vi "Lab Panel V5.22.1.vi"() -> ()   [LabVIEW 2013] (continued)
                    n2885 = Number To Fractional String(number=w5287, precision (6)=w5245) -> (F-format string=w5285:string)  [unwired: 2 in]
                    n2886 = Number To Fractional String(number=w5297, precision (6)=w5245) -> (F-format string=w5295:string)  [unwired: 2 in]
                    n2887 = Number To Fractional String(number=w5292, precision (6)=w5245) -> (F-format string=w5290:string)  [unwired: 2 in]
                    n2888 = Number To Fractional String(number=w5277, precision (6)=w5245) -> (F-format string=w5275:string)  [unwired: 2 in]
                    n2889 = Number To Fractional String(number=w5282, precision (6)=w5245) -> (F-format string=w5280:string)  [unwired: 2 in]
                    n2890 = Number To Fractional String(number=w5307, precision (6)=w5245) -> (F-format string=w5305:string)  [unwired: 2 in]
                    n2891 = Number To Fractional String(number=w5272, precision (6)=w5245) -> (F-format string=w5270:string)  [unwired: 2 in]
                    n2892 = Number To Fractional String(number=w5312, precision (6)=w5245) -> (F-format string=w5310:string)  [unwired: 2 in]
                    n2893 = Number To Fractional String(number=w5314, precision (6)=w5245) -> (F-format string=w5267:string)  [unwired: 2 in]
                    n2894 = Concatenate Strings(w5244, w5286, w5244, w5285, w5244, w5284) -> (w5260:string)
                    n2895 = Concatenate Strings(w5244, w5281, w5244, w5280, w5244, w5279) -> (w5259:string)
                    n2896 = Concatenate Strings(w5244, w5276, w5244, w5275, w5244, w5274) -> (w5258:string)
                    n2897 = Concatenate Strings(w5244, w5271, w5244, w5270, w5244, w5269) -> (w5257:string)
                    n2898 = Concatenate Strings(w5244, w5268, w5244, w5267, w5244, w5266) -> (w5256:string)
                    n2899 = Concatenate Strings(w5244, w5311, w5244, w5310, w5244, w5309) -> (w5265:string)
                    n2900 = Concatenate Strings(w5244, w5291, w5244, w5290, w5244, w5289) -> (w5261:string)
                    n2901 = Concatenate Strings(w5244, w5306, w5244, w5305, w5244, w5304) -> (w5264:string)
                    n2902 = Concatenate Strings(w5244, w5303, w5244, w5302, w5244, w5299) -> (w5263:string)
                    n2903 = Concatenate Strings(w5244, w5296, w5244, w5295, w5244, w5294) -> (w5262:string)
                    n2904 = Concatenate Strings("]", "\r") -> (w5241:string)
                    n2905 = Concatenate Strings(w5236, w5261, w5241) -> (w5251:string)
                    n2906 = Concatenate Strings(w5238, w5263, w5241) -> (w5253:string)
                    n2907 = Concatenate Strings(w5237, w5262, w5241) -> (w5252:string)
                    n2908 = Concatenate Strings(w5233, w5258, w5241) -> (w5248:string)
                    n2909 = Concatenate Strings(w5234, w5257, w5241) -> (w5249:string)
                    n2910 = Concatenate Strings(w5232, w5259, w5241) -> (w5247:string)
                    n2911 = Concatenate Strings(w5231, w5260, w5241) -> (w5246:string)
                    n2912 = Concatenate Strings(w5235, w5256, w5241) -> (w5250:string)
                    n2913 = Concatenate Strings(w5239, w5264, w5241) -> (w5254:string)
                    n2914 = Concatenate Strings(w5240, w5265, w5241) -> (w5255:string)
                    n2915 = Concatenate Strings(w5255, w5254, w5253, w5252, w5251, w5246, w5247, w5248, w5249, w5250) -> (w5224:string)
                    n2916 = Concatenate Strings("[PANEL/", "DESC/", "CYCLES/", "MINS/", "STATUS]", "\r", w5224) -> (w5223:string)
                    "MAIL REPORT" <- w5223
                    n2917 = global write "Global display 3.vi" "log all"(w5223) -> ()
                  }
                  frame #2 {
                    w5354 = "END"
                    n2918 = local read "mail control"() -> (w5355:string)
                    n2919 = case shown="False" w5350 {
                      tunnel: w5355 -> [w5379 _]
                      tunnel: w5354 -> [w5378 _]
                      tunnel: [w5377 FALSE] -> w5340
                      frame False {
                        n2920 = Equal?(x=w5379, y=w5378) -> (x = y?=w5377:bool)
                      }
                      frame True {
                      }
                    }
                    n2921 = case shown="False" w5356 {
                      tunnel: w5355 -> [w5395 _]
                      tunnel: w5354 -> [w5394 _]
                      tunnel: [w5393 FALSE] -> w5344
                      frame False {
                        n2922 = Equal?(x=w5395, y=w5394) -> (x = y?=w5393:bool)
                      }
                      frame True {
                      }
                    }
                    n2923 = case shown="False" w5353 {
                      tunnel: w5355 -> [w5391 _]
                      tunnel: w5354 -> [w5390 _]
                      tunnel: [w5389 FALSE] -> w5343
                      frame False {
                        n2924 = Equal?(x=w5391, y=w5390) -> (x = y?=w5389:bool)
                      }
                      frame True {
                      }
                    }
                    n2925 = case shown="False" w5351 {
                      tunnel: w5355 -> [w5383 _]
                      tunnel: w5354 -> [w5382 _]
                      tunnel: [w5381 FALSE] -> w5341
                      frame False {
                        n2926 = Equal?(x=w5383, y=w5382) -> (x = y?=w5381:bool)
                      }
                      frame True {
                      }
                    }
                    n2927 = case shown="False" w5352 {
                      tunnel: w5355 -> [w5387 _]
                      tunnel: w5354 -> [w5386 _]
                      tunnel: [w5385 FALSE] -> w5342
                      frame False {
                        n2928 = Equal?(x=w5387, y=w5386) -> (x = y?=w5385:bool)
                      }
                      frame True {
                      }
                    }
                    n2929 = Or(x=w5342, y=w5341) -> (x .or. y?=w5333:bool)
                    n2930 = Or(x=w5344, y=w5343) -> (x .or. y?=w5334:bool)
                    n2931 = Or(x=w5334, y=w5333) -> (x .or. y?=w5329:bool)
                    n2932 = case shown="False" w5346 {
                      tunnel: w5355 -> [w5363 _]
                      tunnel: w5354 -> [w5362 _]
                      tunnel: [w5361 FALSE] -> w5335
                      frame False {
                        n2933 = Equal?(x=w5363, y=w5362) -> (x = y?=w5361:bool)
                      }
                      frame True {
                      }
                    }
                    n2934 = case shown="False" w5345 {
                      tunnel: w5355 -> [w5359 _]
                      tunnel: w5354 -> [w5358 _]
                      tunnel: [w5357 FALSE] -> w5339
                      frame False {
                        n2935 = Equal?(x=w5359, y=w5358) -> (x = y?=w5357:bool)
                      }
                      frame True {
                      }
                    }
                    n2936 = case shown="False" w5347 {
                      tunnel: w5355 -> [w5367 _]
                      tunnel: w5354 -> [w5366 _]
                      tunnel: [w5365 FALSE] -> w5336
                      frame False {
                        n2937 = Equal?(x=w5367, y=w5366) -> (x = y?=w5365:bool)
                      }
                      frame True {
                      }
                    }
                    n2938 = case shown="False" w5349 {
                      tunnel: w5355 -> [w5375 _]
                      tunnel: w5354 -> [w5374 _]
                      tunnel: [w5373 FALSE] -> w5338
                      frame False {
                        n2939 = Equal?(x=w5375, y=w5374) -> (x = y?=w5373:bool)
                      }
                      frame True {
                      }
                    }
                    n2940 = case shown="False" w5348 {
                      tunnel: w5355 -> [w5371 _]
                      tunnel: w5354 -> [w5370 _]
                      tunnel: [w5369 FALSE] -> w5337
                      frame False {
                        n2941 = Equal?(x=w5371, y=w5370) -> (x = y?=w5369:bool)
                      }
                      frame True {
                      }
                    }
                    n2942 = Or(x=w5338, y=w5337) -> (x .or. y?=w5332:bool)
                    n2943 = Or(x=w5336, y=w5335) -> (x .or. y?=w5331:bool)
                    n2944 = Or(x=w5339, y=w5340) -> (x .or. y?=w5327:bool)
                    n2945 = Or(x=w5332, y=w5331) -> (x .or. y?=w5330:bool)
                    n2946 = Or(x=w5329, y=w5330) -> (x .or. y?=w5328:bool)
                    n2947 = Or(x=w5328, y=w5327) -> (x .or. y?=w5326:bool)
                  }
                  frame #3 {
                    n2948 = local read "on loops"() -> (w5409:dbl)
                    n2949 = local read "jig cycle"() -> (w5406:dbl)
                    n2950 = local read "Send Mail Now"() -> (w5400:bool)
                    n2951 = Add(x=w5409, y=3.0) -> (x+y=w5407:dbl)
                    n2952 = Equal?(x=w5406, y=w5407) -> (x = y?=w5401:bool)
                    n2953 = And(x=w5401, y=w5400) -> (x .and. y?=w5399:bool)
                    n2954 = And(x=w5405, y=w5401) -> (x .and. y?=w5404:bool)
                    n2955 = And(x=w5404, y=w5403) -> (x .and. y?=w5402:bool)
                    n2956 = Or(x=w5402, y=w5399) -> (x .or. y?=w5398:bool)
                    n2957 = case shown="True" w5398 {
                      tunnel: w5414 -> [_ w5420]
                      tunnel: w5413 -> [_ w5419]
                      tunnel: "Lab Panel Test Status" -> [_ w5418]
                      tunnel: w5411 -> [_ w5417]
                      tunnel: w5410 -> [_ w5416]
                      tunnel: w5397 -> [_ w5415]
                      frame False {
                      }
                      frame True {
                        n2958 = stacked-sequence {
                          tunnel: w5420 -> [w5428 _]
                          tunnel: w5419 -> [w5427 _]
                          tunnel: w5418 -> [w5426 _]
                          tunnel: w5417 -> [w5425 _]
                          tunnel: w5416 -> [w5424 _]
                          tunnel: w5415 -> [w5423 _]
                          frame #0 {
                            n2959 = call "sub vi - send mail v5.vi"("TO:"=w5428, "subject"=w5426, "from"=w5424, "out going server"=w5425, "message"=w5427) -> ("error out"=w5422:errorcluster)  [unwired: 10 in]
                            n2960 = Bundle(cluster=w5423, "mail error"=w5422) -> (w5421:T7)  [unwired: 6 in]
                            n2961 = local write "MAIL SETTINGS"(w5421) -> ()
                          }
                          frame #1 {
                            n2962 = local write "mail control"("") -> ()
                            n2963 = local write "Send Mail Now"(FALSE) -> ()
                          }
                        }
                      }
                    }
                  }
                }
              }
            }
          }
          frame #18 {
            # "save jig cycle values once all run switches are off"
            n2964 = stacked-sequence {
              tunnel: w5440 -> [_ w5469]
              tunnel: w5439 -> [_ w5468]
              tunnel: w5438 -> [_ w5467]
              tunnel: w5437 -> [_ w5466]
              tunnel: w5436 -> [_ w5465]
              tunnel: w5435 -> [_ w5464]
              tunnel: w5434 -> [_ w5463]
              tunnel: w5433 -> [_ w5462]
              tunnel: w5432 -> [_ w5461]
              tunnel: w5431 -> [_ w5460]
              frame #0 {
              }
              frame #1 {
                n2965 = Not(x=w5460) -> (.not. x?=w5443:bool)
                n2966 = Not(x=w5468) -> (.not. x?=w5458:bool)
                n2967 = Not(x=w5465) -> (.not. x?=w5453:bool)
                n2968 = Not(x=w5463) -> (.not. x?=w5449:bool)
                n2969 = Not(x=w5461) -> (.not. x?=w5445:bool)
                n2970 = Not(x=w5469) -> (.not. x?=w5459:bool)
                n2971 = Not(x=w5467) -> (.not. x?=w5457:bool)
                n2972 = Not(x=w5464) -> (.not. x?=w5451:bool)
                n2973 = Not(x=w5466) -> (.not. x?=w5455:bool)
                n2974 = Not(x=w5462) -> (.not. x?=w5447:bool)
                n2975 = local read "Save JC"() -> (w5471:bool)
                n2976 = And(x=w5459, y=w5458) -> (x .and. y?=w5456:bool)
                n2977 = And(x=w5456, y=w5457) -> (x .and. y?=w5454:bool)
                n2978 = And(x=w5454, y=w5455) -> (x .and. y?=w5452:bool)
                n2979 = And(x=w5452, y=w5453) -> (x .and. y?=w5450:bool)
                n2980 = And(x=w5450, y=w5451) -> (x .and. y?=w5448:bool)
                n2981 = And(x=w5448, y=w5449) -> (x .and. y?=w5446:bool)
                n2982 = And(x=w5446, y=w5447) -> (x .and. y?=w5444:bool)
                n2983 = And(x=w5444, y=w5445) -> (x .and. y?=w5442:bool)
                n2984 = And(x=w5442, y=w5443) -> (x .and. y?=w5441:bool)
                n2985 = And(x=w5441, y=w5471) -> (x .and. y?=w5470:bool)
                n2986 = case shown="True" w5470 {
                  tunnel: w5441 -> [w5472 _]
                  frame False {
                    n2987 = case shown="False" w5472 {
                      frame False {
                        n2988 = local write "Save JC"(TRUE) -> ()
                      }
                      frame True {
                      }
                    }
                  }
                  frame True {
                    n2989 = stacked-sequence {
                      frame #0 {
                        n2990 = String To Path(string="c:\\crabtree\\Jig Cycles\\") -> (path=w5484:path)
                        n2991 = Build Path(base path=w5484, name or relative path="jigcycles.bin") -> (appended path=w5482:path)
                        n2992 = Create Folder(path (use dialog)=w5484) -> (error out=w5486:errorcluster)  [unwired: 2 in, 2 out]
                        n2993 = local read "JIG RELAY CYCLES"() -> (w5476:T8)
                        n2994 = call <vilib>:"Clear Errors.vi"("error in (no error)"=w5486) -> ()  [unwired: 6 in, 1 out]
                        n2995 = local write "Save JC"(FALSE) -> ()
                        n2996 = Open/Create/Replace File(file path (use dialog)=w5482, operation (0:open)=T17."replace or create") -> (refnum out=w5480:refnum<file>, error out=w5481:errorcluster)  [unwired: 4 in, 1 out]
                        n2997 = Write to Binary File(file (use dialog)=w5480, data=w5476, error in=w5481) -> (refnum out=w5479:refnum<file>, error out=w5478:errorcluster)  [unwired: 3 in, 1 out]
                        n2998 = Close File(refnum=w5479, error in=w5478) -> (error out=w5477:errorcluster)  [unwired: 1 out]
                        n2999 = local write "data file error"(w5477) -> ()
                      }
                      frame #1 {
                        n3000 = local read "JIG RELAY CYCLES"() -> (w5509:T8)
                        n3001 = Unbundle By Name(w5509) -> ("LAB01-1"=w5504:dbl, "LAB01-2"=w5503:dbl, "LAB02-1"=w5501:dbl, "LAB02-2"=w5500:dbl, "LAB03-1"=w5498:dbl, "LAB03-2"=w5495:dbl, "LAB04-1"=w5494:dbl, "LAB04-2"=w5492:dbl, "LAB05-1"=w5490:dbl, "LAB05-2"=w5488:dbl)
                        n3002 = stacked-sequence {
                          tunnel: w5504 -> [w5512 _ _ _ _ _ _ _ _ _]
                          tunnel: 1000000 -> [w5515 w5525 w5535 w5545 w5555 w5565 w5575 w5585 w5595 w5605]
                          tunnel: [w5513 _ _ _ _ _ _ _ _ _] -> w5507
                          tunnel: "TEST STATION HAS REACHED 1 MILLION CYCLES, REPLACE  CONTROL RELAYS" -> [w5511 w5523 w5533 w5543 w5553 w5563 w5573 w5583 w5593 w5603]
                          tunnel: [_ w5522 _ _ _ _ _ _ _ _] -> w5505
                          tunnel: w5503 -> [_ w5521 _ _ _ _ _ _ _ _]
                          tunnel: [_ _ w5532 _ _ _ _ _ _ _] -> w5502
                          tunnel: w5501 -> [_ _ w5531 _ _ _ _ _ _ _]
                          tunnel: w5500 -> [_ _ _ w5542 _ _ _ _ _ _]
                          tunnel: [_ _ _ w5541 _ _ _ _ _ _] -> w5499
                          tunnel: w5498 -> [_ _ _ _ w5552 _ _ _ _ _]
                          tunnel: [_ _ _ _ w5551 _ _ _ _ _] -> w5497
                          tunnel: [_ _ _ _ _ w5562 _ _ _ _] -> w5496
                          tunnel: w5495 -> [_ _ _ _ _ w5561 _ _ _ _]
                          tunnel: w5494 -> [_ _ _ _ _ _ w5572 _ _ _]
                          tunnel: [_ _ _ _ _ _ w5571 _ _ _] -> w5493
                          tunnel: w5492 -> [_ _ _ _ _ _ _ w5582 _ _]
                          tunnel: [_ _ _ _ _ _ _ w5581 _ _] -> w5491
                          tunnel: w5490 -> [_ _ _ _ _ _ _ _ w5592 _]
                          tunnel: [_ _ _ _ _ _ _ _ w5591 _] -> w5489
                          tunnel: w5488 -> [_ _ _ _ _ _ _ _ _ w5602]
                          tunnel: [_ _ _ _ _ _ _ _ _ w5601] -> w5487
                          frame #0 {
                            n3003 = Greater?(x=w5512, y=w5515) -> (0:w5514:bool)
                            n3004 = case shown="True" w5514 {
                              tunnel: [w5516 0] -> w5513
                              tunnel: w5512 -> [w5516 _]
                              tunnel: w5511 -> [_ w5517]
                              frame False {
                              }
                              frame True {
                                n3005 = Concatenate Strings("LA01-1 ", w5517) -> (w5520:string)
                                n3006 = One Button Dialog(message=w5520) -> ()  [unwired: 1 in, 1 out]
                              }
                            }
                          }
                          frame #1 {
                            n3007 = Greater?(x=w5521, y=w5525) -> (0:w5524:bool)
                            n3008 = case shown="True" w5524 {
                              tunnel: [w5526 0] -> w5522
                              tunnel: w5521 -> [w5526 _]
                              tunnel: w5523 -> [_ w5527]
                              frame False {
                              }
                              frame True {
                                n3009 = Concatenate Strings("LA01-2 ", w5527) -> (w5530:string)
                                n3010 = One Button Dialog(message=w5530) -> ()  [unwired: 1 in, 1 out]
                              }
                            }
                          }
                          frame #2 {
                            n3011 = Greater?(x=w5531, y=w5535) -> (0:w5534:bool)
                            n3012 = case shown="True" w5534 {
                              tunnel: [w5536 0] -> w5532
                              tunnel: w5531 -> [w5536 _]
                              tunnel: w5533 -> [_ w5537]
                              frame False {
                              }
                              frame True {
                                n3013 = Concatenate Strings("LA02-1 ", w5537) -> (w5540:string)
                                n3014 = One Button Dialog(message=w5540) -> ()  [unwired: 1 in, 1 out]
                              }
                            }
                          }
                          frame #3 {
                            n3015 = Greater?(x=w5542, y=w5545) -> (0:w5544:bool)
                            n3016 = case shown="True" w5544 {
                              tunnel: [w5546 0] -> w5541
                              tunnel: w5542 -> [w5546 _]
                              tunnel: w5543 -> [_ w5547]
                              frame False {
                              }
                              frame True {
                                n3017 = Concatenate Strings("LA02-2 ", w5547) -> (w5550:string)
                                n3018 = One Button Dialog(message=w5550) -> ()  [unwired: 1 in, 1 out]
                              }
                            }
                          }
                          frame #4 {
                            n3019 = Greater?(x=w5552, y=w5555) -> (0:w5554:bool)
                            n3020 = case shown="True" w5554 {
                              tunnel: [w5556 0] -> w5551
                              tunnel: w5552 -> [w5556 _]
                              tunnel: w5553 -> [_ w5557]
                              frame False {
                              }
                              frame True {
                                n3021 = Concatenate Strings("LA03-1 ", w5557) -> (w5560:string)
                                n3022 = One Button Dialog(message=w5560) -> ()  [unwired: 1 in, 1 out]
                              }
                            }
                          }
                          frame #5 {
                            n3023 = Greater?(x=w5561, y=w5565) -> (0:w5564:bool)
                            n3024 = case shown="True" w5564 {
                              tunnel: [w5566 0] -> w5562
                              tunnel: w5561 -> [w5566 _]
                              tunnel: w5563 -> [_ w5567]
                              frame False {
                              }
                              frame True {
                                n3025 = Concatenate Strings("LA03-2 ", w5567) -> (w5570:string)
                                n3026 = One Button Dialog(message=w5570) -> ()  [unwired: 1 in, 1 out]
                              }
                            }
                          }
                          frame #6 {
                            n3027 = Greater?(x=w5572, y=w5575) -> (0:w5574:bool)
                            n3028 = case shown="True" w5574 {
                              tunnel: [w5576 0] -> w5571
                              tunnel: w5572 -> [w5576 _]
                              tunnel: w5573 -> [_ w5577]
                              frame False {
                              }
                              frame True {
                                n3029 = Concatenate Strings("LA04-1 ", w5577) -> (w5580:string)
                                n3030 = One Button Dialog(message=w5580) -> ()  [unwired: 1 in, 1 out]
                              }
                            }
                          }
                          frame #7 {
                            n3031 = Greater?(x=w5582, y=w5585) -> (0:w5584:bool)
                            n3032 = case shown="True" w5584 {
                              tunnel: [w5586 0] -> w5581
                              tunnel: w5582 -> [w5586 _]
                              tunnel: w5583 -> [_ w5587]
                              frame False {
                              }
                              frame True {
                                n3033 = Concatenate Strings("LA04-2 ", w5587) -> (w5590:string)
                                n3034 = One Button Dialog(message=w5590) -> ()  [unwired: 1 in, 1 out]
                              }
                            }
                          }
                          frame #8 {
                            n3035 = Greater?(x=w5592, y=w5595) -> (0:w5594:bool)
                            n3036 = case shown="True" w5594 {
                              tunnel: [w5596 0] -> w5591
                              tunnel: w5592 -> [w5596 _]
                              tunnel: w5593 -> [_ w5597]
                              frame False {
                              }
                              frame True {
                                n3037 = Concatenate Strings("LA05-1 ", w5597) -> (w5600:string)
                                n3038 = One Button Dialog(message=w5600) -> ()  [unwired: 1 in, 1 out]
                              }
                            }
                          }
                          frame #9 {
                            n3039 = Greater?(x=w5602, y=w5605) -> (0:w5604:bool)
                            n3040 = case shown="True" w5604 {
                              tunnel: [w5606 0] -> w5601
                              tunnel: w5602 -> [w5606 _]
                              tunnel: w5603 -> [_ w5607]
                              frame False {
                              }
                              frame True {
                                n3041 = Concatenate Strings("LA05-2 ", w5607) -> (w5610:string)
                                n3042 = One Button Dialog(message=w5610) -> ()  [unwired: 1 in, 1 out]
                              }
                            }
                          }
                        }
                        n3043 = Bundle By Name(cluster=w5509, "LAB01-1"=w5507, "LAB01-2"=w5505, "LAB02-1"=w5502, "LAB02-2"=w5499, "LAB03-1"=w5497, "LAB03-2"=w5496, "LAB04-1"=w5493, "LAB04-2"=w5491, "LAB05-1"=w5489, "LAB05-2"=w5487) -> (w5508:T8)
                        n3044 = local write "JIG RELAY CYCLES"(w5508) -> ()
                      }
                    }
                  }
                }
              }
            }
          }
          frame #19 {
            # "get temperature values"
            n3045 = local read "Panel #"() -> (w5611:dbl)
            n3046 = local read "Simulate"() -> (w5624:bool)
            n3047 = local read "Temp Test Cal"() -> (w5621:dbl)
            n3048 = stacked-sequence {
              seq-local: [w5627 _] -> [_ w5720]
              tunnel: w5624 -> [_ w5734]
              tunnel: T14 {"1  (A) cal"=1.0, "1 (V) cal"=1.0, "1 (PF) cal"=1.0, "1 (TL) cal"=1.0, "1 (TN) cal"=1.0, "2 (A) cal"=1.0, "2 (V) cal"=1.0, "2 (PF) cal"=1.0, "2 (TL) cal"=1.0, "2 (TN) cal"=1.0} ("CAL LAB01") -> [_ w5733]
              tunnel: w5622 -> [_ w5732]
              tunnel: w5621 -> [_ w5731]
              tunnel: w5620 -> [_ w5730]
              tunnel: w5619 -> [_ w5729]
              tunnel: w5618 -> [_ w5728]
              tunnel: w5617 -> [_ w5727]
              tunnel: w5616 -> [_ w5726]
              tunnel: w5615 -> [_ w5725]
              tunnel: w5614 -> [_ w5724]
              tunnel: w5613 -> [_ w5723]
              tunnel: w5612 -> [_ w5722]
              tunnel: w5611 -> [_ w5721]
              frame #0 {
                # "only get temperature from initial valid temperature circuits"
                n3049 = local read "Select COM port"() -> (w5628:refnum<visa-resource-name>)
                "COM port" <- w5628
                n3050 = global write "Global 1.vi" "COM port"(w5628) -> ()
                n3051 = global write "Global 1.vi" "tmp dly lps"("Temp Delay Lps") -> ()
                n3052 = global write "Global 1.vi" "dly value"("Temp Value") -> ()
                n3053 = local read "jig cycle"() -> (w5630:dbl)
                n3054 = local read "on loops"() -> (w5632:dbl)
                n3055 = Add(x=w5632, y=3) -> (x+y=w5633:dbl)
                n3056 = local read "Panel #"() -> (w5629:dbl)
                n3057 = Equal?(x=w5630, y=w5633) -> (x = y?=w5627:bool)
                n3058 = stacked-sequence {
                  tunnel: w5629 -> [w5635 _]
                  tunnel: w5627 -> [w5634 _]
                  frame #0 {
                    n3059 = case shown="True" w5634 {
                      tunnel: w5635 -> [_ w5639]
                      frame False {
                      }
                      frame True {
                        n3060 = local read "Simulate"() -> (w5636:bool)
                        n3061 = case shown="5" w5639 {
                          tunnel: 1.0 -> [_ w5642 w5655 w5668 w5680 w5694]
                          tunnel: w5636 -> [_ w5641 w5654 w5667 w5681 w5693]
                          frame 0, Default {
                            (unwired) FALSE
                          }
                          frame 1 {
                            n3062 = local read "LAB01-TP"() -> (w5640:bool)
                            n3063 = case shown="True" w5640 {
                              tunnel: w5642 -> [_ w5652]
                              tunnel: w5641 -> [_ w5648]
                              frame False {
                              }
                              frame True {
                                w5650 = FALSE
                                n3064 = local read "Temp Er 01"() -> (w5645:dbl)
                                n3065 = call "sub vi - GET ALL TEMP v7.vi"("LA01-EN"=TRUE, "simulate"=w5648, "LA02-EN"=w5650, "LA03-EN"=w5650, "LA04-EN"=w5650, "LA05-EN"=w5650, "Gen Cal Value"=w5652) -> ("LA01 TEMP"=w5649:T25, "error"=w5647:bool)  [unwired: 2 in, 5 out]
                                n3066 = Increment(x=w5645) -> (x+1=w5644:dbl)
                                n3067 = local write "LAB01 TEMP"(w5649) -> ()
                                n3068 = Select(t=w5644, s=w5647, f=0.0) -> (s? t:f=→"Temp Er 01":dbl)
                              }
                            }
                          }
                          frame 2 {
                            n3069 = local read "LAB02-TP"() -> (w5653:bool)
                            n3070 = case shown="True" w5653 {
                              tunnel: w5655 -> [_ w5662]
                              tunnel: w5654 -> [_ w5661]
                              frame False {
                              }
                              frame True {
                                w5663 = FALSE
                                n3071 = local read "Temp Er 02"() -> (w5658:dbl)
                                n3072 = call "sub vi - GET ALL TEMP v7.vi"("LA01-EN"=w5663, "simulate"=w5661, "LA02-EN"=TRUE, "LA03-EN"=w5663, "LA04-EN"=w5663, "LA05-EN"=w5663, "Gen Cal Value"=w5662) -> ("LA02 TEMP"=w5665:T25, "error"=w5659:bool)  [unwired: 2 in, 5 out]
                                n3073 = Increment(x=w5658) -> (x+1=w5657:dbl)
                                n3074 = local write "LAB02 TEMP"(w5665) -> ()
                                n3075 = Select(t=w5657, s=w5659, f=0.0) -> (s? t:f=→"Temp Er 02":dbl)
                              }
                            }
                          }
                          frame 3 {
                            n3076 = local read "LAB03-TP"() -> (w5666:bool)
                            n3077 = case shown="True" w5666 {
                              tunnel: w5668 -> [_ w5676]
                              tunnel: w5667 -> [_ w5674]
                              frame False {
                              }
                              frame True {
                                w5677 = FALSE
                                n3078 = local read "Temp Er 03"() -> (w5672:dbl)
                                n3079 = call "sub vi - GET ALL TEMP v7.vi"("LA01-EN"=w5677, "simulate"=w5674, "LA02-EN"=w5677, "LA03-EN"=TRUE, "LA04-EN"=w5677, "LA05-EN"=w5677, "Gen Cal Value"=w5676) -> ("LA03 TEMP"=w5675:T25, "error"=w5670:bool)  [unwired: 2 in, 5 out]
                                n3080 = Increment(x=w5672) -> (x+1=w5671:dbl)
                                n3081 = local write "LAB03 TEMP"(w5675) -> ()
                                n3082 = Select(t=w5671, s=w5670, f=0.0) -> (s? t:f=→"Temp Er 03":dbl)
                              }
                            }
                          }
                          frame 4 {
                            n3083 = local read "LAB04-TP"() -> (w5679:bool)
                            n3084 = case shown="True" w5679 {
                              tunnel: w5681 -> [_ w5689]
                              tunnel: w5680 -> [_ w5688]
                              frame False {
                              }
                              frame True {
                                w5690 = FALSE
                                n3085 = local read "Temp Er 04"() -> (w5686:dbl)
                                n3086 = call "sub vi - GET ALL TEMP v7.vi"("LA01-EN"=w5690, "simulate"=w5689, "LA02-EN"=w5690, "LA03-EN"=w5690, "LA04-EN"=TRUE, "LA05-EN"=w5690, "Gen Cal Value"=w5688) -> ("LA04 TEMP"=w5687:T25, "error"=w5683:bool)  [unwired: 2 in, 5 out]
                                n3087 = Increment(x=w5686) -> (x+1=w5684:dbl)
                                n3088 = local write "LAB04 TEMP"(w5687) -> ()
                                n3089 = Select(t=w5684, s=w5683, f=0.0) -> (s? t:f=→"Temp Er 04":dbl)
                              }
                            }
                          }
                          frame 5 {
                            n3090 = local read "LAB05-TP"() -> (w5692:bool)
                            n3091 = case shown="True" w5692 {
                              tunnel: w5694 -> [_ w5701]
                              tunnel: w5693 -> [_ w5700]
                              frame False {
                              }
                              frame True {
                                w5703 = FALSE
                                n3092 = local read "Temp Er 05"() -> (w5697:dbl)
                                n3093 = call "sub vi - GET ALL TEMP v7.vi"("LA01-EN"=w5703, "simulate"=w5700, "LA02-EN"=w5703, "LA03-EN"=w5703, "LA04-EN"=w5703, "LA05-EN"=TRUE, "Gen Cal Value"=w5701) -> ("error"=w5699:bool, "LA05 TEMP"=w5702:T25)  [unwired: 2 in, 5 out]
                                n3094 = local write "LAB05 TEMP"(w5702) -> ()
                                n3095 = Increment(x=w5697) -> (x+1=w5698:dbl)
                                n3096 = Select(t=w5698, s=w5699, f=0.0) -> (s? t:f=→"Temp Er 05":dbl)
                              }
                            }
                          }
                        }
                        n3097 = local write "TEMP"(TRUE) -> ()
                      }
                    }
                  }
                  frame #1 {
                    w5705 = 5
                    n3098 = local read "Temp Er 05"() -> (w5715:dbl)
                    n3099 = local read "Temp Er 03"() -> (w5717:dbl)
                    n3100 = local read "Temp Er 04"() -> (w5716:dbl)
                    n3101 = local read "Temp Er 01"() -> (w5719:dbl)
                    n3102 = local read "Temp Er 02"() -> (w5718:dbl)
                    n3103 = Greater Or Equal?(x=w5716, y=w5705) -> (x >= y?=w5709:bool)
                    n3104 = Greater Or Equal?(x=w5718, y=w5705) -> (x >= y?=w5711:bool)
                    n3105 = Greater Or Equal?(x=w5717, y=w5705) -> (x >= y?=w5710:bool)
                    n3106 = Greater Or Equal?(x=w5715, y=w5705) -> (x >= y?=w5708:bool)
                    n3107 = Greater Or Equal?(x=w5719, y=w5705) -> (x >= y?=w5712:bool)
                    n3108 = Or(x=w5710, y=w5709) -> (x .or. y?=w5713:bool)
                    n3109 = Or(x=w5712, y=w5711) -> (x .or. y?=w5714:bool)
                    n3110 = Or(x=w5714, y=w5713) -> (x .or. y?=w5707:bool)
                    n3111 = Or(x=w5707, y=w5708) -> (x .or. y?=→"Error Temp":bool)
                  }
                }
              }
              frame #1 {
                n3112 = case shown="True" w5720 {
                  tunnel: w5734 -> [_ w5748]
                  tunnel: w5733 -> [_ w5747]
                  tunnel: w5732 -> [_ w5746]
                  tunnel: w5731 -> [_ w5745]
                  tunnel: w5730 -> [_ w5744]
                  tunnel: w5729 -> [_ w5743]
                  tunnel: w5728 -> [_ w5742]
                  tunnel: w5727 -> [_ w5741]
                  tunnel: w5726 -> [_ w5740]
                  tunnel: w5725 -> [_ w5739]
                  tunnel: w5724 -> [_ w5738]
                  tunnel: w5723 -> [_ w5737]
                  tunnel: w5722 -> [_ w5736]
                  tunnel: w5721 -> [_ w5735]
                  frame False {
                  }
                  frame True {
                    n3113 = case shown="1" w5735 {
                      tunnel: w5748 -> [_ w5761 w5806 w5851 w5896 w5941]
                      tunnel: w5747 -> [_ w5760 w5805 w5850 w5895 w5940]
                      tunnel: w5746 -> [_ w5750 _ _ _ _]
                      tunnel: w5745 -> [_ w5755 w5804 w5849 w5894 w5939]
                      tunnel: w5744 -> [_ w5749 _ _ _ _]
                      tunnel: w5743 -> [_ _ w5795 _ _ _]
                      tunnel: w5742 -> [_ _ w5794 _ _ _]
                      tunnel: w5741 -> [_ _ _ w5840 _ _]
                      tunnel: w5740 -> [_ _ _ w5839 _ _]
                      tunnel: w5739 -> [_ _ _ _ w5885 _]
                      tunnel: w5738 -> [_ _ _ _ w5884 _]
                      tunnel: w5737 -> [_ _ _ _ _ w5930]
                      tunnel: w5736 -> [_ _ _ _ _ w5929]
                      frame ..0 {
                      }
                      frame 1 {
                        n3114 = case shown="False" w5761 {
                          tunnel: [w5792 w5793] -> w5777
                          tunnel: w5760 -> [_ w5793]
                          frame False {
                            n3115 = local read "CAL LAB01"() -> (w5792:T14)
                          }
                          frame True {
                          }
                        }
                        n3116 = local read "TEMP LA01"() -> (w5768:T9)
                        n3117 = local read "LAB01 TEMP"() -> (w5767:T12)
                        n3118 = call "sub vi - temperature delay v3.vi"("2-run"=w5749, "1-run"=w5750, "temp values IN"=w5768, "temp signals"=w5767) -> ("T2-N"=w5763:dbl, "T2-L"=w5764:dbl, "T1-N"=w5765:dbl, "T1-L"=w5766:dbl, "temp values OUT"=w5762:T44)  [unwired: 3 in]
                        n3119 = Unbundle By Name(w5777) -> ("1 (TL) cal"=w5772:dbl, "1 (TN) cal"=w5771:dbl, "2 (TL) cal"=w5770:dbl, "2 (TN) cal"=w5769:dbl)  [unwired: 6 out]
                        n3120 = local write "TEMP LA01"(w5762) -> ()
                        n3121 = Multiply(x=w5766, y=w5772) -> (x*y=w5759:dbl)
                        n3122 = Multiply(x=w5765, y=w5771) -> (x*y=w5757:dbl)
                        n3123 = Multiply(x=w5764, y=w5770) -> (x*y=w5754:dbl)
                        n3124 = Multiply(x=w5763, y=w5769) -> (x*y=w5753:dbl)
                        n3125 = case shown="True" w5750 {
                          tunnel: w5759 -> [w5786 w5791]
                          tunnel: w5755 -> [_ w5789]
                          tunnel: [w5786 w5790] -> w5758
                          tunnel: w5757 -> [w5785 w5788]
                          tunnel: [w5785 w5787] -> w5756
                          frame False {
                          }
                          frame True {
                            n3126 = Multiply(x=w5789, y=w5788) -> (x*y=w5787:dbl)
                            n3127 = Multiply(x=w5789, y=w5791) -> (x*y=w5790:dbl)
                          }
                        }
                        n3128 = case shown="True" w5749 {
                          tunnel: w5754 -> [w5779 w5784]
                          tunnel: w5755 -> [_ w5782]
                          tunnel: [w5779 w5783] -> w5752
                          tunnel: w5753 -> [w5778 w5781]
                          tunnel: [w5778 w5780] -> w5751
                          frame False {
                          }
                          frame True {
                            n3129 = Multiply(x=w5782, y=w5781) -> (x*y=w5780:dbl)
                            n3130 = Multiply(x=w5782, y=w5784) -> (x*y=w5783:dbl)
                          }
                        }
                        n3131 = local read "SIG LAB01-2"() -> (w5774:T2)
                        n3132 = local read "SIG LAB01-1"() -> (w5776:T2)
                        n3133 = Bundle By Name(cluster=w5776, "Tmp Live"=w5758, "Tmp Neut"=w5756) -> (w5775:T2)
                        n3134 = Bundle By Name(cluster=w5774, "Tmp Live"=w5752, "Tmp Neut"=w5751) -> (w5773:T2)
                        n3135 = local write "SIG LAB01-1"(w5775) -> ()
                        n3136 = local write "SIG LAB01-2"(w5773) -> ()
                      }
                      frame 2 {
                        n3137 = case shown="True" w5806 {
                          tunnel: [w5837 w5838] -> w5822
                          tunnel: w5805 -> [_ w5838]
                          frame False {
                            n3138 = local read "CAL LAB02"() -> (w5837:T15)
                          }
                          frame True {
                          }
                        }
                        n3139 = local read "LAB02 TEMP"() -> (w5813:T12)
                        n3140 = local read "TEMP LA02"() -> (w5812:T9)
                        n3141 = call "sub vi - temperature delay v3.vi"("2-run"=w5794, "1-run"=w5795, "temp values IN"=w5812, "temp signals"=w5813) -> ("T2-N"=w5807:dbl, "T2-L"=w5808:dbl, "T1-N"=w5809:dbl, "T1-L"=w5810:dbl, "temp values OUT"=w5811:T44)  [unwired: 3 in]
                        n3142 = Unbundle By Name(w5822) -> ("1 (TL) cal"=w5817:dbl, "1 (TN) cal"=w5816:dbl, "2 (TL) cal"=w5815:dbl, "2 (TN) cal"=w5814:dbl)  [unwired: 6 out]
                        n3143 = local write "TEMP LA02"(w5811) -> ()
                        n3144 = Multiply(x=w5810, y=w5817) -> (x*y=w5803:dbl)
                        n3145 = Multiply(x=w5809, y=w5816) -> (x*y=w5802:dbl)
                        n3146 = Multiply(x=w5808, y=w5815) -> (x*y=w5799:dbl)
                        n3147 = Multiply(x=w5807, y=w5814) -> (x*y=w5798:dbl)
                        n3148 = case shown="True" w5795 {
                          tunnel: w5803 -> [w5831 w5836]
                          tunnel: w5804 -> [_ w5834]
                          tunnel: [w5831 w5835] -> w5801
                          tunnel: w5802 -> [w5830 w5833]
                          tunnel: [w5830 w5832] -> w5800
                          frame False {
                          }
                          frame True {
                            n3149 = Multiply(x=w5834, y=w5833) -> (x*y=w5832:dbl)
                            n3150 = Multiply(x=w5834, y=w5836) -> (x*y=w5835:dbl)
                          }
                        }
                        n3151 = case shown="True" w5794 {
                          tunnel: w5799 -> [w5824 w5829]
                          tunnel: w5804 -> [_ w5827]
                          tunnel: [w5824 w5828] -> w5797
                          tunnel: w5798 -> [w5823 w5826]
                          tunnel: [w5823 w5825] -> w5796
                          frame False {
                          }
                          frame True {
                            n3152 = Multiply(x=w5827, y=w5826) -> (x*y=w5825:dbl)
                            n3153 = Multiply(x=w5827, y=w5829) -> (x*y=w5828:dbl)
                          }
                        }
                        n3154 = local read "SIG LAB02-2"() -> (w5819:T2)
                        n3155 = local read "SIG LAB02-1"() -> (w5821:T2)
                        n3156 = Bundle By Name(cluster=w5821, "Tmp Live"=w5801, "Tmp Neut"=w5800) -> (w5820:T2)
                        n3157 = Bundle By Name(cluster=w5819, "Tmp Live"=w5797, "Tmp Neut"=w5796) -> (w5818:T2)
                        n3158 = local write "SIG LAB02-1"(w5820) -> ()
                        n3159 = local write "SIG LAB02-2"(w5818) -> ()
                      }
                      frame 3 {
                        n3160 = case shown="False" w5851 {
                          tunnel: [w5882 w5883] -> w5867
                          tunnel: w5850 -> [_ w5883]
                          frame False {
                            n3161 = local read "CAL LAB03"() -> (w5882:T14)
                          }
                          frame True {
                          }
                        }
                        n3162 = local read "TEMP LA03"() -> (w5857:T9)
                        n3163 = local read "LAB03 TEMP"() -> (w5858:T12)
                        n3164 = call "sub vi - temperature delay v3.vi"("2-run"=w5839, "1-run"=w5840, "temp values IN"=w5857, "temp signals"=w5858) -> ("T2-N"=w5852:dbl, "T2-L"=w5853:dbl, "T1-N"=w5854:dbl, "T1-L"=w5855:dbl, "temp values OUT"=w5856:T44)  [unwired: 3 in]
                        n3165 = Unbundle By Name(w5867) -> ("1 (TL) cal"=w5862:dbl, "1 (TN) cal"=w5861:dbl, "2 (TL) cal"=w5860:dbl, "2 (TN) cal"=w5859:dbl)  [unwired: 6 out]
                        n3166 = local write "TEMP LA03"(w5856) -> ()
                        n3167 = Multiply(x=w5855, y=w5862) -> (x*y=w5848:dbl)
                        n3168 = Multiply(x=w5854, y=w5861) -> (x*y=w5847:dbl)
                        n3169 = Multiply(x=w5853, y=w5860) -> (x*y=w5844:dbl)
                        n3170 = Multiply(x=w5852, y=w5859) -> (x*y=w5843:dbl)
                        n3171 = case shown="True" w5839 {
                          tunnel: w5844 -> [w5869 w5874]
                          tunnel: w5849 -> [_ w5872]
                          tunnel: [w5869 w5873] -> w5842
                          tunnel: w5843 -> [w5868 w5871]
                          tunnel: [w5868 w5870] -> w5841
                          frame False {
                          }
                          frame True {
                            n3172 = Multiply(x=w5872, y=w5871) -> (x*y=w5870:dbl)
                            n3173 = Multiply(x=w5872, y=w5874) -> (x*y=w5873:dbl)
                          }
                        }
                        n3174 = case shown="True" w5840 {
                          tunnel: w5848 -> [w5876 w5881]
                          tunnel: w5849 -> [_ w5879]
                          tunnel: [w5876 w5880] -> w5846
                          tunnel: w5847 -> [w5875 w5878]
                          tunnel: [w5875 w5877] -> w5845
                          frame False {
                          }
                          frame True {
                            n3175 = Multiply(x=w5879, y=w5878) -> (x*y=w5877:dbl)
                            n3176 = Multiply(x=w5879, y=w5881) -> (x*y=w5880:dbl)
                          }
                        }
                        n3177 = local read "SIG LAB03-2"() -> (w5864:T2)
                        n3178 = local read "SIG LAB03-1"() -> (w5866:T2)
                        n3179 = Bundle By Name(cluster=w5866, "Tmp Live"=w5846, "Tmp Neut"=w5845) -> (w5865:T2)
                        n3180 = Bundle By Name(cluster=w5864, "Tmp Live"=w5842, "Tmp Neut"=w5841) -> (w5863:T2)
                        n3181 = local write "SIG LAB03-1"(w5865) -> ()
                        n3182 = local write "SIG LAB03-2"(w5863) -> ()
                      }
                      frame 4 {
                        n3183 = case shown="False" w5896 {
                          tunnel: [w5927 w5928] -> w5912
                          tunnel: w5895 -> [_ w5928]
                          frame False {
                            n3184 = local read "CAL LAB04"() -> (w5927:T14)
                          }
                          frame True {
                          }
                        }
                        n3185 = local read "LAB04 TEMP"() -> (w5902:T12)
                        n3186 = local read "TEMP LA04"() -> (w5903:T9)
                        n3187 = call "sub vi - temperature delay v3.vi"("2-run"=w5884, "1-run"=w5885, "temp values IN"=w5903, "temp signals"=w5902) -> ("T2-N"=w5897:dbl, "T2-L"=w5898:dbl, "T1-N"=w5899:dbl, "T1-L"=w5900:dbl, "temp values OUT"=w5901:T44)  [unwired: 3 in]
                        n3188 = Unbundle By Name(w5912) -> ("1 (TL) cal"=w5907:dbl, "1 (TN) cal"=w5906:dbl, "2 (TL) cal"=w5905:dbl, "2 (TN) cal"=w5904:dbl)  [unwired: 6 out]
                        n3189 = local write "TEMP LA04"(w5901) -> ()
                        n3190 = Multiply(x=w5900, y=w5907) -> (x*y=w5893:dbl)
                        n3191 = Multiply(x=w5899, y=w5906) -> (x*y=w5892:dbl)
                        n3192 = Multiply(x=w5898, y=w5905) -> (x*y=w5889:dbl)
                        n3193 = Multiply(x=w5897, y=w5904) -> (x*y=w5888:dbl)
                        n3194 = case shown="True" w5884 {
                          tunnel: w5889 -> [w5914 w5919]
                          tunnel: w5894 -> [_ w5917]
                          tunnel: [w5914 w5918] -> w5887
                          tunnel: w5888 -> [w5913 w5916]
                          tunnel: [w5913 w5915] -> w5886
                          frame False {
                          }
                          frame True {
                            n3195 = Multiply(x=w5917, y=w5916) -> (x*y=w5915:dbl)
                            n3196 = Multiply(x=w5917, y=w5919) -> (x*y=w5918:dbl)
                          }
                        }
                        n3197 = case shown="True" w5885 {
                          tunnel: w5893 -> [w5921 w5926]
                          tunnel: w5894 -> [_ w5924]
                          tunnel: [w5921 w5925] -> w5891
                          tunnel: w5892 -> [w5920 w5923]
                          tunnel: [w5920 w5922] -> w5890
                          frame False {
                          }
                          frame True {
                            n3198 = Multiply(x=w5924, y=w5923) -> (x*y=w5922:dbl)
                            n3199 = Multiply(x=w5924, y=w5926) -> (x*y=w5925:dbl)
                          }
                        }
                        n3200 = local read "SIG LAB04-2"() -> (w5909:T2)
                        n3201 = local read "SIG LAB04-1"() -> (w5911:T2)
                        n3202 = Bundle By Name(cluster=w5911, "Tmp Live"=w5891, "Tmp Neut"=w5890) -> (w5910:T2)
                        n3203 = Bundle By Name(cluster=w5909, "Tmp Live"=w5887, "Tmp Neut"=w5886) -> (w5908:T2)
                        n3204 = local write "SIG LAB04-1"(w5910) -> ()
                        n3205 = local write "SIG LAB04-2"(w5908) -> ()
                      }
                      frame 5.. {
                        n3206 = case shown="False" w5941 {
                          tunnel: [w5972 w5973] -> w5957
                          tunnel: w5940 -> [_ w5973]
                          frame False {
                            n3207 = local read "CAL LAB05"() -> (w5972:T14)
                          }
                          frame True {
